vi "NXT_MIDBRAIN Right Wall Follow Behavior Data.vi"(1 "_sensorData":T2={"_irData"={"_irDistance"=0, "_irHeading"=0, "_irTimestamp"=0}, "_batteryVoltage"=0, "_NXTButtonStates"=[FALSE, FALSE, FALSE]}, 2 "Behavior #":i32, 3 "Previous Motor Position":T1={"_rudderCommand"=7, "_propCommand"=7, "_irServoCommand"=7}, 4 "Behavior Weights":T4=[0, 0, 0, 0, 0, 0]) -> (0 "Behavior Output":T5)   [LabVIEW 2012]
uses:
  behaviorOutput_t.ctl
  behaviorWeights_t.ctl
  sensorData_t.ctl
  irData_t.ctl
  motorCommands_t.ctl
panel:
  # "L\nE\nF\nT"
  # "C\nE\nN\nT\nE\nR"
  # "R\nI\nG\nH\nT"
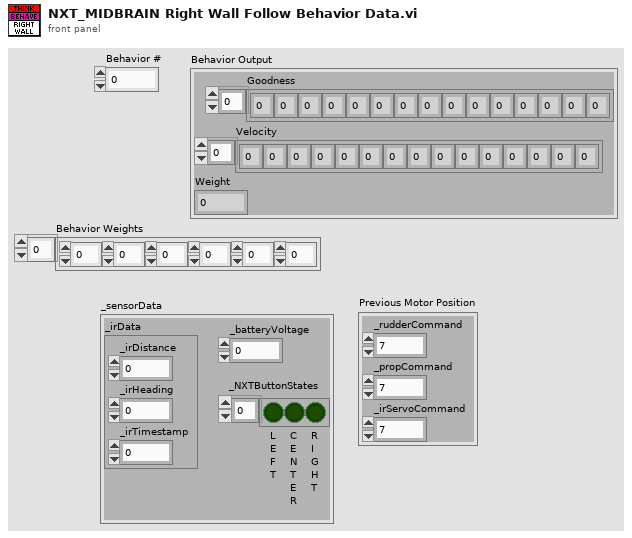
[diagram p1: front panel]
types:
  T1 = typedef "motorCommands_t.ctl" = cluster{"_rudderCommand":i8, "_propCommand":i8, "_irServoCommand":i8}
  T2 = typedef "sensorData_t.ctl" = cluster{"_irData":T3, "_batteryVoltage":i32, "_NXTButtonStates":bool[]}
  T3 = typedef "irData_t.ctl" = cluster{"_irDistance":i32, "_irHeading":i32, "_irTimestamp":u32}
  T4 = typedef "behaviorWeights_t.ctl" = i8[]
  T5 = typedef "behaviorOutput_t.ctl" = cluster{"Goodness":i8[], "Velocity":i8[], "Weight":i8}
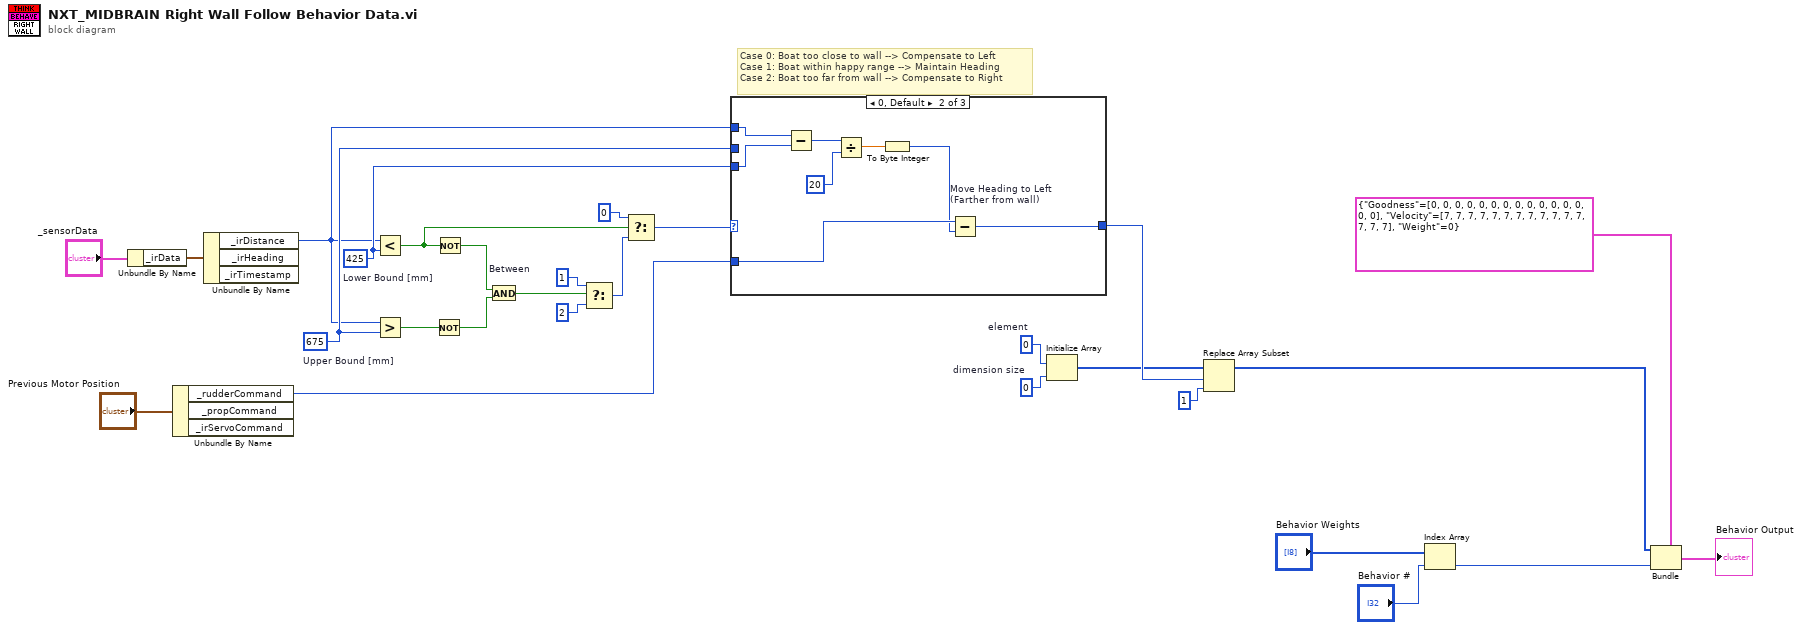
[diagram p0: block diagram]
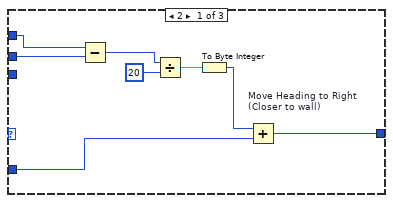
[diagram p2: hidden frame]
diagram:
  w3 = 0  # dimension size
  w4 = i8 0  # element
  w9 = 675  # Upper Bound [mm]
  w8 = 425  # Lower Bound [mm]
  # "Case 0: Boat too close to wall --> Compensate to Left\nCase 1: Boat within happy range --> Maintain Heading\nCase 2: Boat too far from wall --> Compensate to Right"
  n1 = Unbundle By Name("_sensorData") -> ("_irData"=w22:T3)
  n2 = Unbundle By Name("Previous Motor Position") -> ("_rudderCommand"=w10:i8)  [unwired: 2 out]
  n3 = Unbundle By Name(w22) -> ("_irDistance"=w7:i32)  [unwired: 2 out]
  n4 = Less?(x=w7, y=w8) -> (x < y?=w19:bool)
  n5 = Greater?(x=w7, y=w9) -> (0:w16:bool)
  n6 = Not(x=w16) -> (.not. x?=w20:bool)
  n7 = Not(x=w19) -> (.not. x?=w21:bool)
  n8 = And "Between"(x=w21, y=w20) -> (x .and. y?=w18:bool)
  n9 = Select(t=1, s=w18, f=2) -> (s? t:f=w17:i32)
  n10 = Select(t=0, s=w19, f=w17) -> (s? t:f=w12:i32)
  n11 = case shown="0, Default" w12 {
    tunnel: w10 -> [w29 w38 w45]
    tunnel: [w31 w42 w45] -> w6
    tunnel: w9 -> [w35 _ _]
    tunnel: w8 -> [_ w43 _]
    tunnel: w7 -> [w36 w44 _]
    frame 2 {
      n12 = Subtract(x=w36, y=w35) -> (x-y=w34:i8)
      n13 = Divide(x=w34, y=i8 20) -> (x/y=w32:dbl)
      n14 = To Byte Integer(number=w32) -> (8bit integer=w30:i8)
      n15 = Add "Move Heading to Right\n(Closer to wall)"(x=w30, y=w29) -> (x+y=w31:i8)
    }
    frame 0, Default {
      n16 = Subtract(x=w44, y=w43) -> (x-y=w41:i32)
      n17 = Divide(x=w41, y=20) -> (x/y=w39:dbl)
      n18 = To Byte Integer(number=w39) -> (8bit integer=w37:i8)
      n19 = Subtract "Move Heading to Left\n(Farther from wall)"(x=w38, y=w37) -> (x-y=w42:i8)
    }
    frame 1 {
    }
  }
  n20 = Initialize Array(w4, w3) -> (w2:i8[])
  n21 = Replace Array Subset(array=w2, new element=i8 1 ("new element/subarray"), index=w6) -> (w1:i8[])
  n22 = Index Array(array="Behavior Weights", index="Behavior #") -> (element=w24:i8)
  n23 = Bundle(cluster=T5 {"Goodness"=[0, 0, 0, 0, 0, 0, 0, 0, 0, 0, 0, 0, 0, 0, 0], "Velocity"=[7, 7, 7, 7, 7, 7, 7, 7, 7, 7, 7, 7, 7, 7, 7], "Weight"=0} ("Behavior Output"), "Goodness"=w1, "Weight"=w24) -> (→"Behavior Output":T5)  [unwired: 1 in]
